vi "MMME P01 SubVI03.vi"(3 "D":bool, 5 "C":bool, 7 "B":bool, 11 "A":bool) -> (0 "h":bool, 1 "d":bool, 2 "b":bool, 4 "g":bool, 6 "f":bool, 8 "e":bool, 9 "c":bool, 10 "a":bool)   [LabVIEW 2021]
doc: "Este programa permite la transferencia de datos correspondiente al SUBVI principal, ya que, con este convertidor de BCD nos ayuda con lo realizado en el SUBVI interno obteniendo al final el programa completo\n- Creador: Mendoza Meza Manuel Everardo\n- Grupo: 3MV5\n- Periodo: 2022/2"
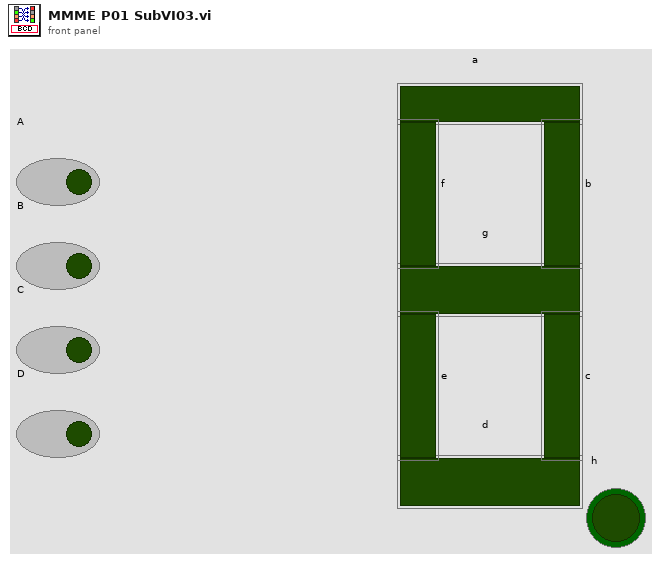
[diagram p1: front panel]
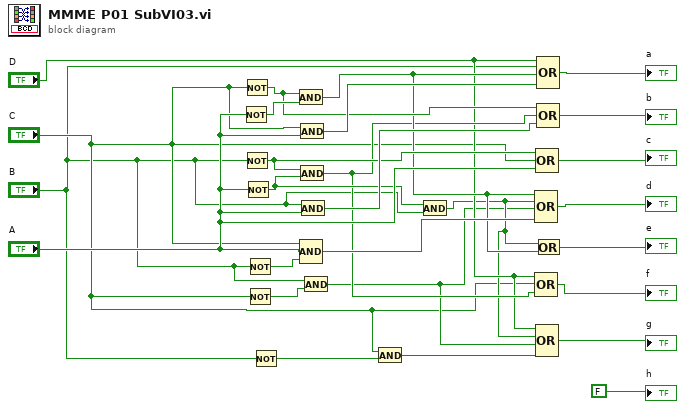
[diagram p0: block diagram]
diagram:
  n1 = Not(x="A") -> (.not. x?=w25:bool)
  n2 = Not(x="C") -> (.not. x?=w21:bool)
  n3 = Not(x="B") -> (.not. x?=w20:bool)
  n4 = Not(x="A") -> (.not. x?=w14:bool)
  n5 = Not(x="B") -> (.not. x?=w16:bool)
  n6 = Not(x="C") -> (.not. x?=w4:bool)
  n7 = Not(x="B") -> (.not. x?=w2:bool)
  n8 = And(x=w21, y=w25) -> (x .and. y?=w12:bool)
  n9 = And(x="C", y="A") -> (x .and. y?=w24:bool)
  n10 = And(x=w20, y=w14) -> (x .and. y?=w10:bool)
  n11 = And(x="B", y="A") -> (x .and. y?=w22:bool)
  n12 = Compound Arithmetic op=AND("C", "A", w16) -> (w15:bool)
  n13 = And(x="B", y=w4) -> (x .and. y?=w6:bool)
  n14 = And(x="C", y=w2) -> (x .and. y?=w5:bool)
  n15 = And(x=w14, y="B") -> (x .and. y?=w7:bool)
  n16 = Or(x=w7, y=w12) -> (x .or. y?=→"e":bool)
  n17 = Compound Arithmetic op=OR(w12, w7, w6, w15) -> (→"d":bool)
  n18 = Compound Arithmetic op=OR("D", "C", w10) -> (→"f":bool)
  n19 = Compound Arithmetic op=OR(w20, "C", "A") -> (→"c":bool)
  n20 = Compound Arithmetic op=OR("D", w7, w6, w5) -> (→"g":bool)
  n21 = Compound Arithmetic op=OR("D", "B", w12, w24) -> (→"a":bool)
  n22 = Compound Arithmetic op=OR(w21, w10, w22) -> (→"b":bool)
  "h" <- FALSE
